vi "rest arm from starting position.vi"   [LabVIEW 2018]
types:
  T1 = enum16{"shoulder", "elbow", "wrist", "base", "gripper"}
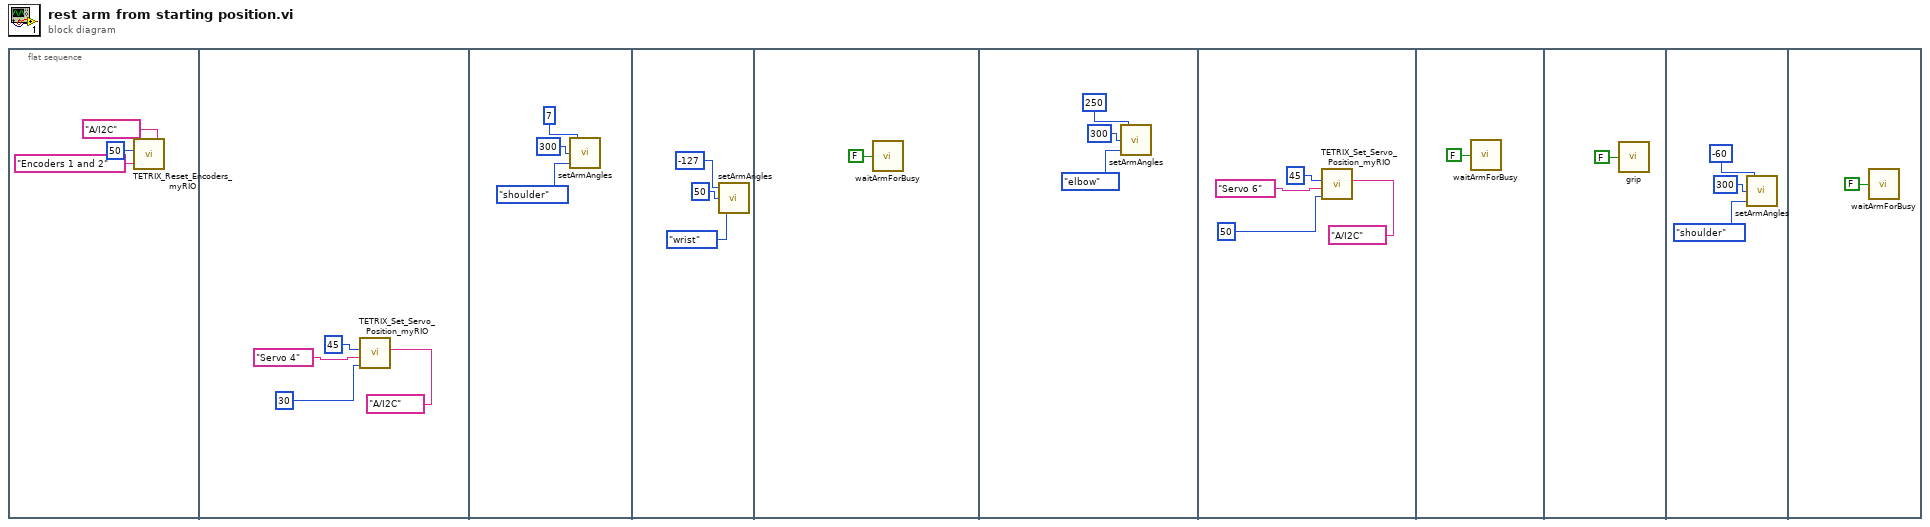
[diagram p0: block diagram]
diagram:
  n1 = flat-sequence {
    frame #0 {
      n2 = call <vilib>:"TETRIX_Reset_Encoders_myRIO.vi"("myRIO MXP Port A/B"=tag "A/I2C", "Select Encoder"="Encoders 1 and 2", "Controller ID#  (I2C Address)"=u8 50) -> ()  [unwired: 4 in, 1 out]
    }
    frame #1 {
      n3 = call <vilib>:"TETRIX_Set_Servo_Position_myRIO.vi"("myRIO MXP Port A/B"=tag "A/I2C", "Set Servo Position (0 - 180 degrees)"=u8 30, "Select Channel"="Servo 4", "Controller ID#  (I2C Address)"=u8 45) -> ()  [unwired: 3 in, 1 out]
    }
    frame #2 {
      n4 = call "setArmAngles.vi"("Enum"=T1."shoulder", "speed"=300, "angle"=7) -> ()  [unwired: 1 in]
    }
    frame #3 {
      n5 = call "setArmAngles.vi"("Enum"=T1."wrist", "speed"=50, "angle"=-127) -> ()  [unwired: 1 in]
    }
    frame #4 {
      n6 = call "waitArmForBusy.vi"("base"=FALSE) -> ()
    }
    frame #5 {
      n7 = call "setArmAngles.vi"("Enum"=T1."elbow", "speed"=300, "angle"=250) -> ()  [unwired: 1 in]
    }
    frame #6 {
      n8 = call <vilib>:"TETRIX_Set_Servo_Position_myRIO.vi"("myRIO MXP Port A/B"=tag "A/I2C", "Set Servo Position (0 - 180 degrees)"=u8 50 ("Set Servo Position (0 - 180 degrees) 2"), "Select Channel"="Servo 6", "Controller ID#  (I2C Address)"=u8 45) -> ()  [unwired: 3 in, 1 out]
    }
    frame #7 {
      n9 = call "waitArmForBusy.vi"("base"=FALSE) -> ()
    }
    frame #8 {
      n10 = call "grip.vi"("grip"=FALSE) -> ()
    }
    frame #9 {
      n11 = call "setArmAngles.vi"("Enum"=T1."shoulder", "speed"=300, "angle"=-60) -> ()  [unwired: 1 in]
    }
    frame #10 {
      n12 = call "waitArmForBusy.vi"("base"=FALSE) -> ()
    }
  }
